vi "Dummy Instance VI.vi"(2 "clone#":i32) -> ()   [LabVIEW 2020, in "NI_TargetHelper.lvlib"]
uses:
  <vilib>/TargetSupport/NI_TargetHelper/NI_TargetHelper.lvlib
panel:
  # "allow optional config cluster input\nallow optional summary cluster output\nadd clone# to uniquify channels\n   (e.g., if target is in re-entrant VI each subVI call\n    needs distinct channels)"
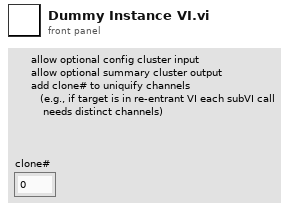
[diagram p1: front panel]
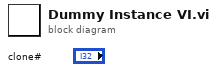
[diagram p0: block diagram]
diagram:
